vi "GetEmptyCatchIndex.vi"(6 "Right Block":bool, 7 "Left Block":bool, 8 "Up Color":i16, 9 "Down Color":i16, 10 "Catch Color":dbl[](array[numeric])) -> (0 "Do Not Thing":bool, 2 "Empty Catch Index":i16)   [LabVIEW 2018]
panel:
  in  "Use Table":bool
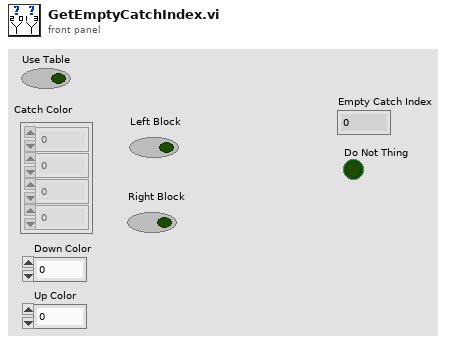
[diagram p1: front panel]
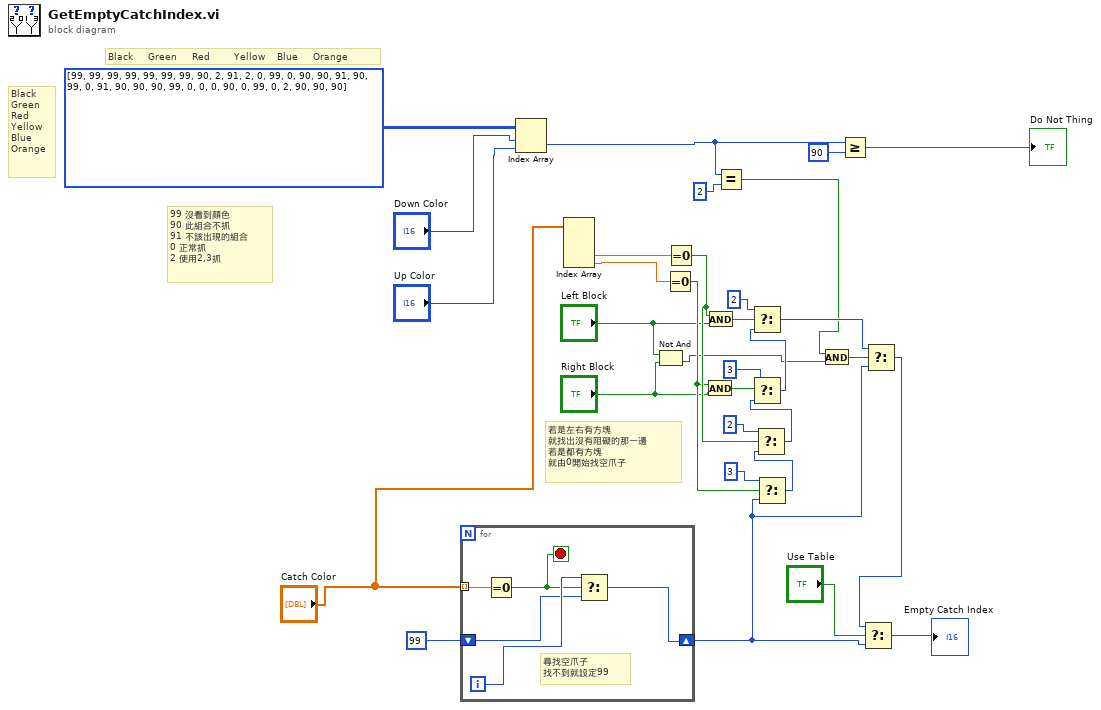
[diagram p0: block diagram]
diagram:
  # "若是左右有方塊\n就找出沒有阻礙的那一邊\n若是都有方塊\n就由0開始找空爪子"
  # "99 沒看到顏色\n90 此組合不抓\n91 不該出現的組合\n0 正常抓\n2 使用2,3抓"
  # "Black\nGreen\nRed\nYellow\nBlue\nOrange"
  # "Black     Green     Red        Yellow    Blue     Orange"
  n1 = for {
    tunnel: "Catch Color" -> [w37] mode=indexing
    shift-right: [w33] -> w9
    shift-left: 99 -> [w35]
    i -> [w36]
    stop <- w34 stop-if-true
    # "尋找空爪子\n找不到就設定99"
    n2 = Equal To 0?(x=w37) -> (x = 0?=w34:bool)
    n3 = Select(t=w36, s=w34, f=w35) -> (s? t:f=w33:i32)
  }
  n4 = Index Array(array=i32[][] [[99, 99, 99, 99, 99, 99], [99, 90, 2, 91, 2, 0], [99, 0, 90, 90, 91, 90], [99, 0, 91, 90, 90, 90], [99, 0, 0, 0, 90, 0], [99, 0, 2, 90, 90, 90]], index (row)="Down Color", index (col)="Up Color") -> (element=w11:i32)
  n5 = Index Array(array="Catch Color") -> (element #3=w27:dbl, element #4=w26:dbl)  [unwired: 4 in, 2 out]
  n6 = Not And(1:"Right Block", 2:"Left Block") -> (0:w1:bool)
  n7 = Equal To 0?(x=w26) -> (x = 0?=w19:bool)
  n8 = Equal To 0?(x=w27) -> (x = 0?=w20:bool)
  n9 = And(x=w19, y="Right Block") -> (x .and. y?=w24:bool)
  n10 = And(x=w20, y="Left Block") -> (x .and. y?=w25:bool)
  n11 = Equal?(x=w11, y=i16 2 ("t")) -> (x = y?=w2:bool)
  n12 = Select(t=i16 3, s=w19, f=w9) -> (s? t:f=w16:i32)
  n13 = Select(t=i16 2, s=w20, f=w16) -> (s? t:f=w15:i32)
  n14 = Select(t=i16 3, s=w24, f=w15) -> (s? t:f=w21:i32)
  n15 = Select(t=i16 2, s=w25, f=w21) -> (s? t:f=w10:i32)
  n16 = And(x=w2, y=w1) -> (x .and. y?=w3:bool)
  n17 = Greater Or Equal?(x=w11, y=90) -> (x >= y?=→"Do Not Thing":bool)
  n18 = Select(t=w10, s=w3, f=w9) -> (s? t:f=w8:i32)
  n19 = Select(t=w8, s="Use Table", f=w9) -> (s? t:f=→"Empty Catch Index":i32)
